vi "gentec-SOLO_PE.Open Connection.vi"(4 "error in":errorcluster, 7 "VISA resource name in":refnum<visa-resource-name>) -> (0 "error out":errorcluster, 2 "Error":string, 3 "VISA resource name out":refnum<visa-resource-name>)   [LabVIEW 2014, in "gentec-SOLO-PE - Driver.lvlib"]
doc: "This VI opens a VISA connection and sets several attributes."
uses:
  gentec-SOLO-PE - Driver.lvlib
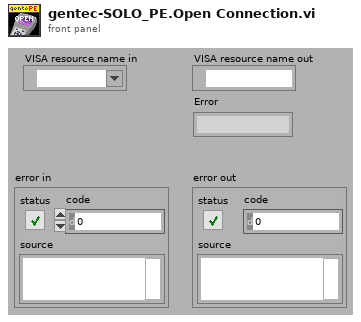
[diagram p1: front panel]
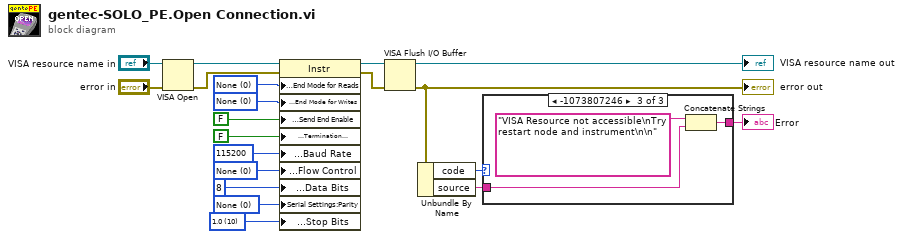
[diagram p0: block diagram]
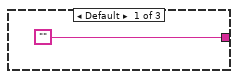
[diagram p2: hidden frame]
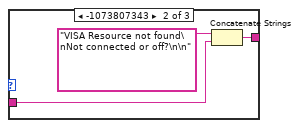
[diagram p3: hidden frame]
diagram:
  w6 = u16 10 items=["1.0"=10, "1.5"=15, "2.0"=20] ("Serial Settings:Stop Bits")
  w7 = u16 0 items=["None", "Odd", "Even", "Mark", "Space"] ("Serial Settings:Parity")
  w9 = u16 0 items=["None"=0, "XON/XOFF"=1, "RTS/CTS"=2, "DTR/DSR"=4] ("Serial Settings:Serial Flow Control")
  w13 = u16 0 items=["None", "LastBit", "TermChar"] ("Serial Settings:Serial End Mode for Reads")
  w14 = u16 0 items=["None", "LastBit", "TermChar", "Break"] ("Serial Settings:Serial End Mode for Writes")
  n1 = VISA Open(error in (no error)="error in", VISA resource name="VISA resource name in") -> (VISA resource name=w18:refnum<visa-resource-name>, error out=w17:errorcluster)  [unwired: 3 in]
  n2 = property class="Instr"(reference=w18, error in=w17, "Serial Settings:End Mode for Reads"=w13, "Serial Settings:End Mode for Writes"=w14, "Message Based Settings:Send End Enable"=FALSE, "Message Based Settings:Termination Character Enable"=FALSE, "Serial Settings:Baud Rate"=u32 115200, "Serial Settings:Flow Control"=w9, "Serial Settings:Data Bits"=u16 8, "Serial Settings:Parity"=w7, "Serial Settings:Stop Bits"=w6) -> (reference out=w12:refnum<visa-resource-name>, error out=w11:errorcluster)
  n3 = VISA Flush I/O Buffer(VISA resource name=w12, error in (no error)=w11) -> (VISA resource name out=→"VISA resource name out":refnum<visa-resource-name>, error out=w2:errorcluster)  [unwired: 1 in]
  "error out" <- w2
  n4 = Unbundle By Name(w2) -> ("code"=w4:i32, "source"=w3:string)
  n5 = case shown="-1073807246" w4 {
    tunnel: w3 -> [_ w24 w27]
    tunnel: ["" w22 w25] -> w1
    frame Default {
    }
    frame -1073807343 {
      n6 = Concatenate Strings("VISA Resource not found\nNot connected or off?\n\n" ("string"), w24) -> (w22:string)
    }
    frame -1073807246 {
      n7 = Concatenate Strings("VISA Resource not accessible\nTry restart node and instrument\n\n" ("string"), w27) -> (w25:string)
    }
  }
  "Error" <- w1
